vi "17.3 OCR.vi"() -> ()   [LabVIEW 2017]
doc: "This example shows how to use the optical character recognition (OCR) VIs in NI Vision. OCR is the process by which a machine vision application reads text and/or characters in inspection images. First, use the OCR Training Interface to teach your application the characters you want to read. The OCR Training Interface creates an OCR session file, which you then use to read characters that you have learned."
uses:
  <vilib>/vision/OCR.llb/IMAQ OCR Character Report 2.ctl
  <vilib>/vision/NI_Vision_Development_Module.lvlib
panel:
  out "Character Reports":T1[](array[typedef]) {"Character Statistics"."Threshold Range"."Upper value" format="%.2f"; "Character Statistics"."Threshold Range"."Lower value" format="%.2f"}
  in  "Stop":bool
  in  "Delay (s.)":dbl(slide)=0.5079365079365079 scale=0.0..2.0
  out "Image":T2(plugin-control)
  out "License Nr.":string
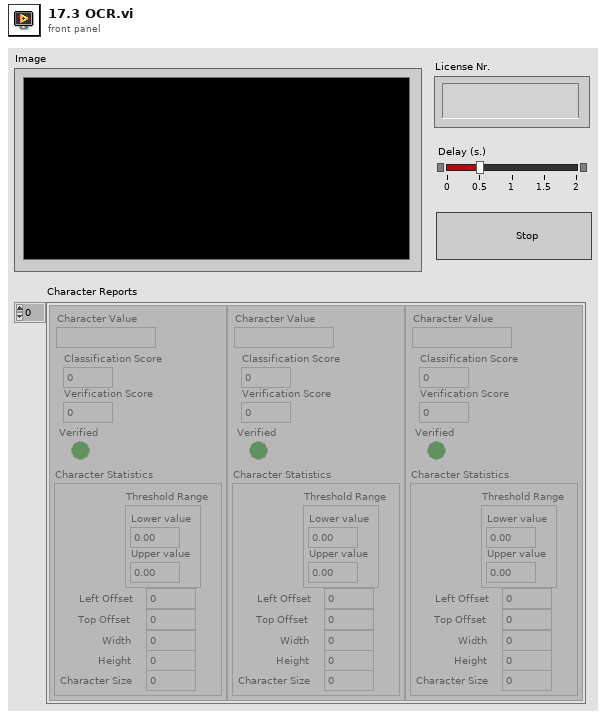
[diagram p1: front panel]
types:
  T1 = typedef "IMAQ OCR Character Report 2.ctl" = cluster{"Character Value":string, "Classification Score":i32, "Verification Score":i32, "Verified":bool, "Character Statistics":cluster{"Threshold Range":cluster{"Lower value":sgl, "Upper value":sgl}, "Left Offset":i32, "Top Offset":i32, "Width":i32, "Height":i32, "Character Size":i32}}
  T2 = typedef "IMAQ Image.ctl" = refnum<image>
  T3 = typedef "IMAQ Rectangle" = cluster{"Left":i32, "Top":i32, "Right":i32, "Bottom":i32, "Rotation":dbl}
  T4 = typedef "IMAQ OCR Session.ctl" = refnum<k1>
  T5 = typedef "ROI Descriptor" = cluster{"Global Rectangle":i32[], "Contours":cluster{"ID":enum32{"External", "Internal"}, "Type":u32, "Coordinates":i32[]}[]}
  T6 = cluster{"Global Rectangle":i32[], "Contours":cluster{"ID":enum32{"External", "Internal"}, "Type":u32, "Coordinates":i32[]}[]}
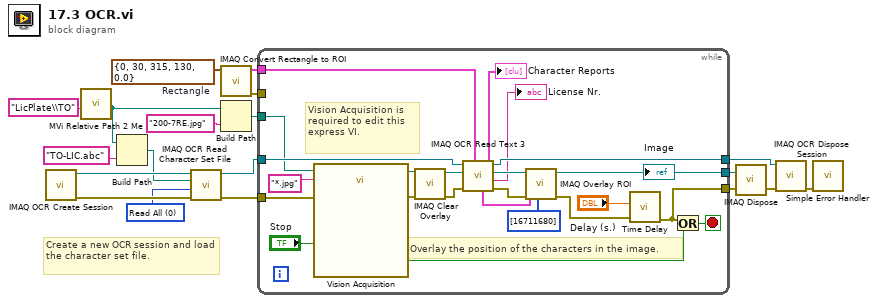
[diagram p0: block diagram]
diagram:
  w14 = T3 {"Left"=0, "Top"=30, "Right"=315, "Bottom"=130, "Rotation"=0.0}  # Rectangle
  w15 = 0 items=["Read All", "Read Character Set Only", "Read Properties Only"] ("Read Options")
  # "Create a new OCR session and load the character set file."
  n1 = call "IMAQ OCR Create Session"() -> ("error out"=w17:errorcluster, "IMAQ OCR Session"=w18:T4)  [unwired: 1 in, 9 out]
  n2 = call "MVi Relative Path 2 Me.vi"("Relative Path"="LicPlate\\TO") -> ("Appended Dir"=w2:path)  [unwired: 5 in, 1 out]
  n3 = Build Path(base path=w2, name or relative path="TO-LIC.abc") -> (appended path=w16:path)
  n4 = call "IMAQ OCR Read Character Set File"("File Path"=w16, "error in (no error)"=w17, "Read Options"=w15, "IMAQ OCR Session"=w18) -> ("error out"=w8:errorcluster, "IMAQ OCR Session (dup)"=w19:T4)  [unwired: 1 in, 5 out]
  n5 = call "IMAQ Convert Rectangle to ROI"("Rectangle"=w14) -> ("error out"=w1:errorcluster, "ROI Descriptor"=w13:T5)  [unwired: 8 in]
  n6 = Build Path(base path=w2, name or relative path="200-7RE.jpg") -> (appended path=w9:path)
  n7 = while {
    tunnel: w13 -> [w41]
    tunnel: w19 -> [w42]
    tunnel: [w28] -> w12
    tunnel: [w37] -> w7
    tunnel: [w27] -> w11
    tunnel: w9 -> [w26]
    tunnel: w8 -> [w21]
    tunnel: w1 -> [_]
    stop <- w33 stop-if-true
    # "Vision Acquisition is required to edit this express VI."
    # "Overlay the position of the characters in the image."
    n8 = call "Vision Acquisition"("Image Path"=w26, "Image File Type (All Types)"="*.jpg", "Stop (F)"="Stop", "error in"=w21) -> ("Image Out"=w32:T2, "Stopped"=w25:bool, "error out"=w30:errorcluster)  [unwired: 21 in]
    n9 = call "IMAQ Clear Overlay"("error in (no error)"=w30, "Image"=w32) -> ("error out"=w23:errorcluster, "Image Out"=w31:T2)  [unwired: 1 in, 7 out]
    n10 = call "IMAQ OCR Read Text 3"("ROI Descriptor"=w41, "error in (no error)"=w23, "Image"=w31, "IMAQ OCR Session"=w42) -> ("error out"=w22:errorcluster, "Read String"=→"License Nr.":string, "Image (dup)"=w38:T2, "IMAQ OCR Session (dup)"=w37:T4, "ROI Bounding Characters"=w40:T6, "Character Reports"=→"Character Reports":T1[])  [unwired: 1 in, 1 out]
    n11 = call "IMAQ Overlay ROI"("Colors (Green)"=u32[] [16711680], "error in (no error)"=w22, "ROI Descriptor"=w40, "Image"=w38) -> ("error out"=w35:errorcluster, "Image Out"=w28:T2)  [unwired: 2 in, 4 out]
    "Image" <- w28
    n12 = call "Time Delay"("error in (no error)"=w35, "Delay Time (s)"="Delay (s.)") -> ("error out"=w27:errorcluster)  [unwired: 9 in]
    n13 = Or(x=w27, y=w25) -> (x .or. y?=w33:bool)
  }
  n14 = call "IMAQ Dispose"("Image"=w12, "error in (no error)"=w11) -> ("error out"=w5:errorcluster)  [unwired: 1 in, 3 out]
  n15 = call "IMAQ OCR Dispose Session"("error in (no error)"=w5, "IMAQ OCR Session"=w7) -> ("error out"=w6:errorcluster)  [unwired: 9 out]
  n16 = call <vilib>:"Simple Error Handler.vi"("error in (no error)"=w6) -> ()  [unwired: 4 in, 5 out]
